vi "Ime Nemo_Register lenght(0).vi"(8 "Array U16":u16[](array[numeric])) -> (0 "Cluster":T2 {"Sys current" format="%.1p"; "Sys voltage" format="%.1p"; "Cosphi" format="%.1p"; "Frequenza" format="%.1p"; "Energia attiva -" format="%.2f"; "Energia attiva +" format="%.2f"; "Tensione FN3" format="%.1p"; "Tensione FN2" format="%.1p"; "Tensione FN1" format="%.1p"; "Papparente" format="%.2f"; "Preattiva" format="%.2f"; "Corrente 3" format="%.3f"; "Corrente 2" format="%.3f"; "TensioneL31" format="%.1p"; "TensioneL23" format="%.1p"; "TensioneL12" format="%.1p"; "Corrente" format="%.3f"; "Pattiva" format="%.2f"}, 3 "Cluster 2":T1 {"Deviation from average of currents [I1,I2,I3]" format="%.2f"; "Deviation from average of voltages [U1,U2,U3]" format="%.2f"; "Maximum deviation from average of currents" format="%.2f"; "Maximum deviation from average of voltages" format="%.2f"; "Phase angle voltage U3-U1" format="%.2f"; "Phase angle voltage U2-U3" format="%.2f"; "Phase angle voltage U1-U2" format="%.2f"; "Average value of currents (I1+I2+I3)/3" format="%.2f"; "Average value of voltages (U1x+U2x+U3x)/3" format="%.2f"; "Load factor phase 3 (L3 – N)" format="%.2f"; "Load factor phase 2 (L2 – N)" format="%.2f"; "Load factor phase 1 (L1 – N)" format="%.2f"; "sign(Q)·(1 – abs(PF)), Load factor system" format="%.2f"; "Reactive power factor phase 1 (L3 – N)" format="%.2f"; "Reactive power factor phase 1 (L2 – N)" format="%.2f"; "Reactive power factor phase 1 (L1 – N)" format="%.2f"; "QF = Q / S, Reactive power factor system" format="%.2f"; "Power factor phase 3 (L3 – N)" format="%.2f"; "Power factor phase 2 (L2 – N)" format="%.2f"; "Power factor phase 1 (L1 – N)" format="%.2f"; "PF = P / S, Power factor system PF" format="%.2f"; "System frequency" format="%.2f"; "Apparent power phase 3 (L3 – N)" format="%.2f"; "Apparent power phase 2 (L2 – N)" format="%.2f"; "Apparent power phase 1 (L1 – N)" format="%.2f"; "Apparent power system S" format="%.2f"; "Reactive power phase 3 (L3 – N)" format="%.2f"; "Reactive power phase 2 (L2 – N)" format="%.2f"; "Reactive power phase 1 (L1 – N)" format="%.2f"; "Reactive power system (Q = Q1 + Q2 + Q3)" format="%.2f"; "Active power phase 3 (L3 – N)" format="%.2f"; "Active power phase 2 (L2 – N)" format="%.2f"; "Active power phase 1 (L1 – N)" format="%.2f"; "Active power system (P = P1 + P2 + P3)" format="%.2f"; "Bimetal current in phase L3" format="%.2f"; "Bimetal current in phase L2" format="%.2f"; "Bimetal current in phase L 1" format="%.2f"; "Bimet curr in balan load sys" format="%.2f"; "Neutral current" format="%.2f"; "Current in phase L3" format="%.2f"; "Current in phase L2" format="%.2f"; "Current in phase L1" format="%.2f"; "System current" format="%.2f"; "Zero displac volt 4w sys" format="%.2f"; "Voltage phase L3 to L1" format="%.2f"; "Voltage phase L2 to L3" format="%.2f"; "Voltage phase L1 to L2" format="%.2f"; "Voltage phase L3 to N" format="%.2f"; "Voltage phase L2 to N" format="%.2f"; "Voltage phase L1 to N" format="%.2f"; "System voltage" format="%.2f"})   [LabVIEW 2019]
panel:
  out "data":dbl[](array[numeric])
  out "Operating time counter":u16
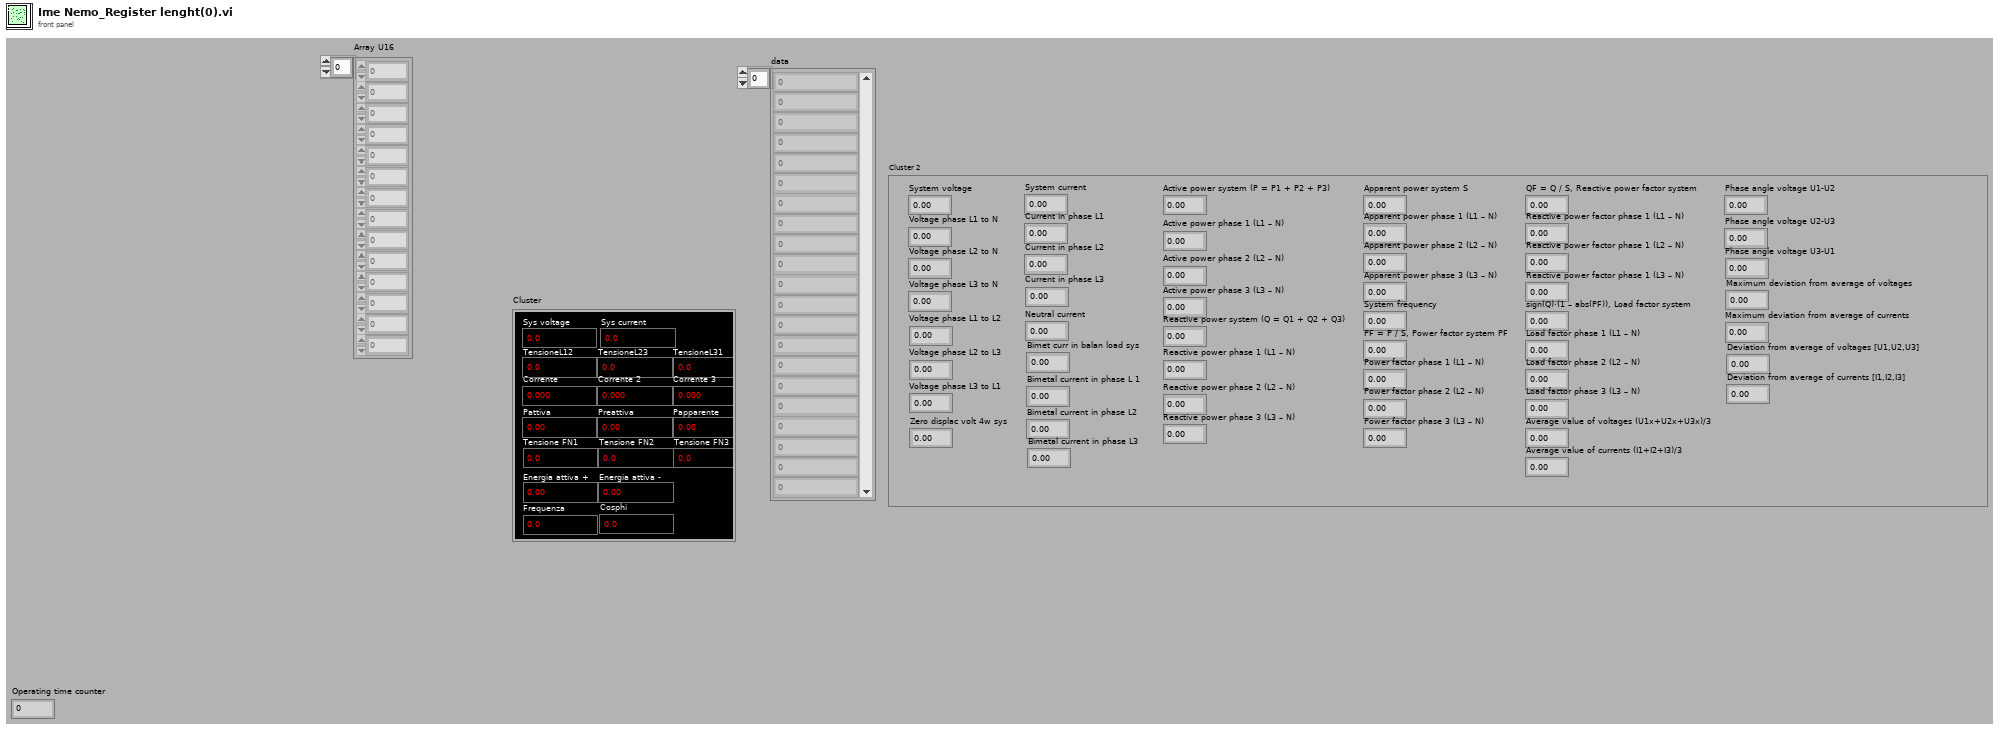
[diagram p1: front panel]
types:
  T1 = cluster{"System voltage":dbl, "Voltage phase L1 to N":dbl, "Voltage phase L2 to N":dbl, "Voltage phase L3 to N":dbl, "Voltage phase L1 to L2":dbl, "Voltage phase L2 to L3":dbl, "Voltage phase L3 to L1":dbl, "Zero displac volt 4w sys":dbl, "System current":dbl, "Current in phase L1":dbl, "Current in phase L2":dbl, "Current in phase L3":dbl, "Neutral current":dbl, "Bimet curr in balan load sys":dbl, "Bimetal current in phase L 1":dbl, "Bimetal current in phase L2":dbl, "Bimetal current in phase L3":dbl, "Active power system (P = P1 + P2 + P3)":dbl, "Active power phase 1 (L1 – N)":dbl, "Active power phase 2 (L2 – N)":dbl, "Active power phase 3 (L3 – N)":dbl, "Reactive power system (Q = Q1 + Q2 + Q3)":dbl, "Reactive power phase 1 (L1 – N)":dbl, "Reactive power phase 2 (L2 – N)":dbl, "Reactive power phase 3 (L3 – N)":dbl, "Apparent power system S":dbl, "Apparent power phase 1 (L1 – N)":dbl, "Apparent power phase 2 (L2 – N)":dbl, "Apparent power phase 3 (L3 – N)":dbl, "System frequency":dbl, "PF = P / S, Power factor system PF":dbl, "Power factor phase 1 (L1 – N)":dbl, "Power factor phase 2 (L2 – N)":dbl, "Power factor phase 3 (L3 – N)":dbl, "QF = Q / S, Reactive power factor system":dbl, "Reactive power factor phase 1 (L1 – N)":dbl, "Reactive power factor phase 1 (L2 – N)":dbl, "Reactive power factor phase 1 (L3 – N)":dbl, "sign(Q)·(1 – abs(PF)), Load factor system":dbl, "Load factor phase 1 (L1 – N)":dbl, "Load factor phase 2 (L2 – N)":dbl, "Load factor phase 3 (L3 – N)":dbl, "Average value of voltages (U1x+U2x+U3x)/3":dbl, "Average value of currents (I1+I2+I3)/3":dbl, "Phase angle voltage U1-U2":dbl, "Phase angle voltage U2-U3":dbl, "Phase angle voltage U3-U1":dbl, "Maximum deviation from average of voltages":dbl, "Maximum deviation from average of currents":dbl, "Deviation from average of voltages [U1,U2,U3]":dbl, "Deviation from average of currents [I1,I2,I3]":dbl}
  T2 = cluster{"Pattiva":dbl, "Corrente":dbl, "TensioneL12":dbl, "TensioneL23":dbl, "TensioneL31":dbl, "Corrente 2":dbl, "Corrente 3":dbl, "Preattiva":dbl, "Papparente":dbl, "Tensione FN1":dbl, "Tensione FN2":dbl, "Tensione FN3":dbl, "Energia attiva +":dbl, "Energia attiva -":dbl, "Frequenza":dbl, "Cosphi":dbl, "Sys voltage":dbl, "Sys current":dbl}
  T3 = cluster{"[0]":dbl, "[1]":dbl, "[2]":dbl, "[3]":dbl, "[4]":dbl, "[5]":dbl, "[6]":dbl, "[7]":dbl, "[8]":dbl, "[9]":dbl, "[10]":dbl, "[11]":dbl, "[12]":dbl, "[13]":dbl, "[14]":dbl, "[15]":dbl, "[16]":dbl, "[17]":dbl, "[18]":dbl, "[19]":dbl, "[20]":dbl, "[21]":dbl, "[22]":dbl, "[23]":dbl, "[24]":dbl, "[25]":dbl, "[26]":dbl, "[27]":dbl, "[28]":dbl, "[29]":dbl, "[30]":dbl, "[31]":dbl, "[32]":dbl, "[33]":dbl, "[34]":dbl, "[35]":dbl, "[36]":dbl, "[37]":dbl, "[38]":dbl, "[39]":dbl, "[40]":dbl, "[41]":dbl, "[42]":dbl, "[43]":dbl, "[44]":dbl, "[45]":dbl, "[46]":dbl, "[47]":dbl, "[48]":dbl, "[49]":dbl, "[50]":dbl}
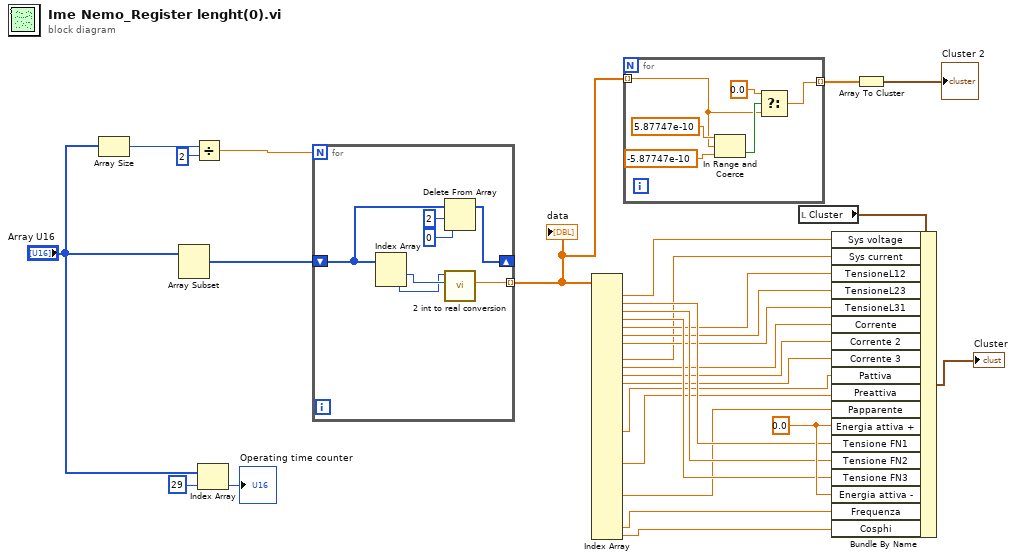
[diagram p0: block diagram]
diagram:
  w24 = 0.0 ("Energia attiva +")
  n1 = Array Size(array="Array U16") -> (size(s)=w22:i32)
  n2 = Array Subset(array="Array U16") -> (w29:u16[])  [unwired: 2 in]
  n3 = Divide(x=w22, y=2) -> (x/y=w28:dbl)
  n4 = Index Array(array="Array U16", index=29) -> (element=→"Operating time counter":u16)
  n5 = for {
    N: w28 -> [_]
    shift-right: [w35] -> _
    shift-left: w29 -> [w36]
    tunnel: [w34] -> w2 mode=indexing
    n6 = Index Array(array=w36) -> (element #1=w31:u16, element #2=w30:u16)  [unwired: 2 in]
    n7 = Delete From Array(array=w36, length=2, index=0) -> (array with subset deleted=w35:u16[])  [unwired: 1 out]
    n8 = call "2 int to real conversion.vi"("MW 15 0 in"=w31, "MW 31 16 in"=w30) -> ("reale out"=w34:dbl)  [unwired: 7 in, 2 out]
  }
  "data" <- w2
  n9 = Index Array(array=w2) -> (element #1=w5:dbl, element #2=w21:dbl, element #3=w20:dbl, element #4=w19:dbl, element #5=w18:dbl, element #6=w17:dbl, element #7=w16:dbl, element #9=w4:dbl, element #10=w15:dbl, element #11=w14:dbl, element #12=w13:dbl, element #18=w12:dbl, element #22=w11:dbl, element #26=w10:dbl, element #30=w8:dbl, element #31=w9:dbl)  [unwired: 31 in, 15 out]
  n10 = for {
    tunnel: w2 -> [w37] mode=indexing
    tunnel: [w42] -> w1 mode=indexing
    n11 = In Range and Coerce(upper limit=5.87747e-10 ("y"), x=w37, lower limit=-5.87747e-10 ("y")) -> (In Range?=w39:bool)  [unwired: 1 out]
    n12 = Select(t=0.0 ("f"), s=w39, f=w37) -> (s? t:f=w42:dbl)
  }
  n13 = local read "Cluster"() -> (w6:T2)
  n14 = Bundle By Name(cluster=w6, "Sys voltage"=w5, "Sys current"=w4, "TensioneL12"=w18, "TensioneL23"=w17, "TensioneL31"=w16, "Corrente"=w15, "Corrente 2"=w14, "Corrente 3"=w13, "Pattiva"=w12, "Preattiva"=w11, "Papparente"=w10, "Energia attiva +"=w24, "Tensione FN1"=w21, "Tensione FN2"=w20, "Tensione FN3"=w19, "Energia attiva -"=w24, "Frequenza"=w8, "Cosphi"=w9) -> (→"Cluster":T2)
  n15 = Array To Cluster(array=w1) -> (cluster=→"Cluster 2":T3)
